vi "Find_All_References.vi"(6 "error in":errorcluster) -> (0 "error out":errorcluster, 1 "INI References":T1(array[cluster]), 2 "CTL References":T1(array[cluster]), 3 "VI References":T1(array[cluster]), 4 "Global References":T1(array[cluster]))   [LabVIEW 2021]
uses:
  Project_References_Global.vi
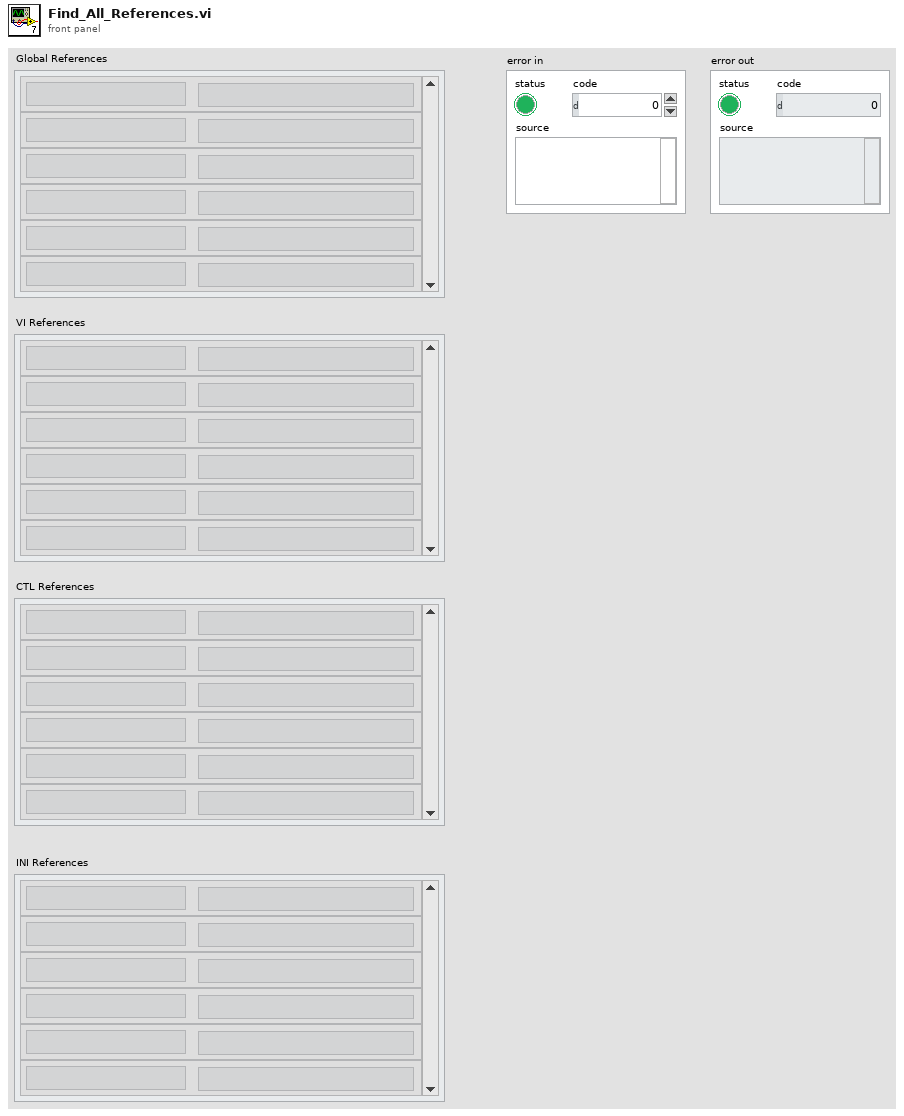
[diagram p1: front panel]
types:
  T1 = cluster{"VI Name":string, "String Path":string}[]
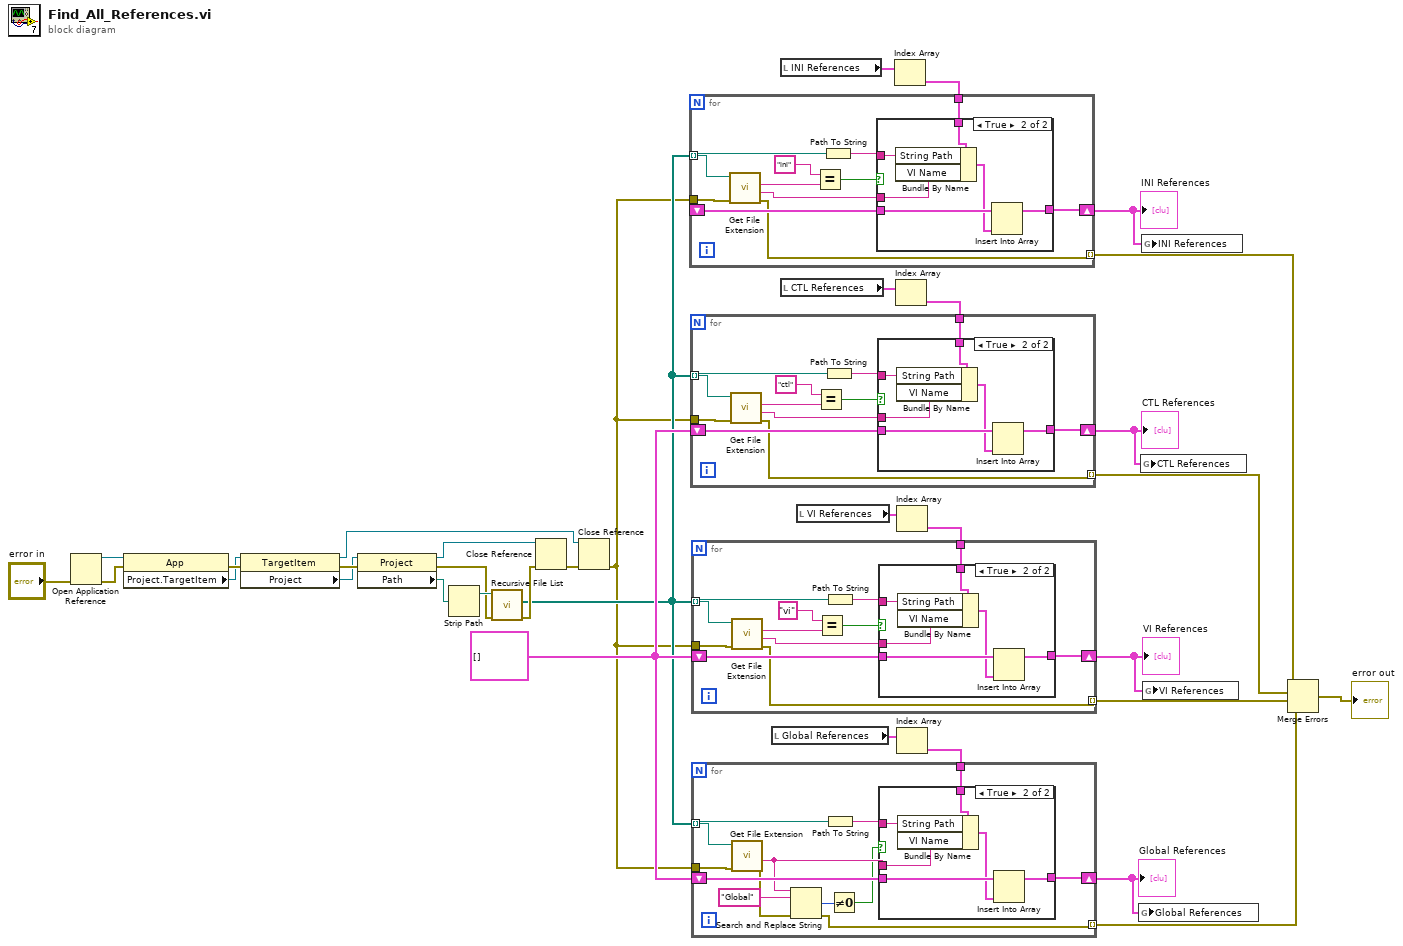
[diagram p0: block diagram]
diagram:
  w17 = T1 [] ("References")
  n1 = Open Application Reference(8:"error in") -> (0:w33:errorcluster, 3:w34:refnum<vi>)  [unwired: 3 in]
  n2 = property class="App"(reference=w34, error in=w33) -> (error out=w32:errorcluster, "Project.TargetItem"=w26:refnum<vi>)  [unwired: 1 out]
  n3 = property class="TargetItem"(reference=w26, error in=w32) -> (reference out=w27:refnum<vi>, error out=w31:errorcluster, "Project"=w30:refnum<vi>)
  n4 = property class="Project"(reference=w30, error in=w31) -> (reference out=w29:refnum<vi>, error out=w13:errorcluster, "Path"=w25:path)
  n5 = Strip Path(path=w25) -> (stripped path=w24:path)  [unwired: 1 out]
  n6 = call <vilib>:"Recursive File List.vi"("error in (no error)"=w13, "Folder Path"=w24) -> ("error out"=w12:errorcluster, "All Files in Dir"=w3:path[])  [unwired: 5 in, 3 out]
  n7 = Close Reference(reference=w29, error in (no error)=w12) -> (error out=w28:errorcluster)
  n8 = Close Reference(reference=w27, error in (no error)=w28) -> (error out=w2:errorcluster)
  n9 = local read "Global References"() -> (w20:T1)
  n10 = local read "INI References"() -> (w5:T1)
  n11 = local read "CTL References"() -> (w18:T1)
  n12 = local read "VI References"() -> (w23:T1)
  n13 = Index Array(array=w5) -> (element=w4:cluster{"VI Name":string, "String Path":string})  [unwired: 1 in]
  n14 = for {
    tunnel: w3 -> [w37] mode=indexing
    tunnel: w4 -> [w45]
    shift-right: [w39] -> w6
    shift-left: _ -> [w40]
    tunnel: w2 -> [w36]
    tunnel: [w35] -> w1 mode=indexing
    n15 = call <vilib>:"Get File Extension.vi"("error in (no error)"=w36, "file"=w37) -> ("error out"=w35:errorcluster, "filename without extension"=w41:string, "lowercase file extension"=w44:string)  [unwired: 5 in, 2 out]
    n16 = Equal?(x="ini", y=w44) -> (x = y?=w42:bool)
    n17 = Path To String(path=w37) -> (string=w38:string)
    n18 = case shown="True" w42 {
      tunnel: w45 -> [_ w52]
      tunnel: w41 -> [_ w51]
      tunnel: w38 -> [_ w50]
      tunnel: w40 -> [w46 w49]
      tunnel: [w46 w48] -> w39
      frame False {
      }
      frame True {
        n19 = Bundle By Name(cluster=w52, "String Path"=w50, "VI Name"=w51) -> (w47:cluster{"VI Name":string, "String Path":string})
        n20 = Insert Into Array(array=w49, new element=w47) -> (w48:T1)  [unwired: 1 in]
      }
    }
  }
  "INI References" <- w6
  n21 = Index Array(array=w18) -> (element=w19:cluster{"VI Name":string, "String Path":string})  [unwired: 1 in]
  n22 = for {
    tunnel: w3 -> [w55] mode=indexing
    tunnel: w19 -> [w63]
    shift-right: [w57] -> w16
    shift-left: w17 -> [w58]
    tunnel: w2 -> [w54]
    tunnel: [w53] -> w11 mode=indexing
    n23 = call <vilib>:"Get File Extension.vi"("error in (no error)"=w54, "file"=w55) -> ("error out"=w53:errorcluster, "filename without extension"=w59:string, "lowercase file extension"=w62:string)  [unwired: 5 in, 2 out]
    n24 = Equal?(x="ctl", y=w62) -> (x = y?=w60:bool)
    n25 = Path To String(path=w55) -> (string=w56:string)
    n26 = case shown="True" w60 {
      tunnel: w63 -> [_ w70]
      tunnel: w59 -> [_ w69]
      tunnel: w56 -> [_ w68]
      tunnel: w58 -> [w64 w67]
      tunnel: [w64 w66] -> w57
      frame False {
      }
      frame True {
        n27 = Bundle By Name(cluster=w70, "String Path"=w68, "VI Name"=w69) -> (w65:cluster{"VI Name":string, "String Path":string})
        n28 = Insert Into Array(array=w67, new element=w65) -> (w66:T1)  [unwired: 1 in]
      }
    }
  }
  "CTL References" <- w16
  n29 = Index Array(array=w23) -> (element=w22:cluster{"VI Name":string, "String Path":string})  [unwired: 1 in]
  n30 = for {
    tunnel: w3 -> [w73] mode=indexing
    tunnel: w22 -> [w81]
    shift-right: [w75] -> w15
    shift-left: w17 -> [w76]
    tunnel: w2 -> [w72]
    tunnel: [w71] -> w10 mode=indexing
    n31 = call <vilib>:"Get File Extension.vi"("error in (no error)"=w72, "file"=w73) -> ("error out"=w71:errorcluster, "filename without extension"=w77:string, "lowercase file extension"=w80:string)  [unwired: 5 in, 2 out]
    n32 = Equal?(x="vi", y=w80) -> (x = y?=w78:bool)
    n33 = Path To String(path=w73) -> (string=w74:string)
    n34 = case shown="True" w78 {
      tunnel: w81 -> [_ w88]
      tunnel: w77 -> [_ w87]
      tunnel: w74 -> [_ w86]
      tunnel: w76 -> [w82 w85]
      tunnel: [w82 w84] -> w75
      frame False {
      }
      frame True {
        n35 = Bundle By Name(cluster=w88, "String Path"=w86, "VI Name"=w87) -> (w83:cluster{"VI Name":string, "String Path":string})
        n36 = Insert Into Array(array=w85, new element=w83) -> (w84:T1)  [unwired: 1 in]
      }
    }
  }
  "VI References" <- w15
  n37 = Index Array(array=w20) -> (element=w21:cluster{"VI Name":string, "String Path":string})  [unwired: 1 in]
  n38 = for {
    tunnel: w3 -> [w96] mode=indexing
    tunnel: w21 -> [w100]
    shift-right: [w98] -> w14
    shift-left: w17 -> [w99]
    tunnel: w2 -> [w91]
    tunnel: [w89] -> w9 mode=indexing
    n39 = call <vilib>:"Get File Extension.vi"("error in (no error)"=w91, "file"=w96) -> ("error out"=w90:errorcluster, "filename without extension"=w95:string)  [unwired: 5 in, 3 out]
    n40 = Search and Replace String(input string=w95, search string="Global", error in=w90) -> (number of replacements=w93:i32, error out=w89:errorcluster)  [unwired: 5 in, 2 out]
    n41 = Path To String(path=w96) -> (string=w97:string)
    n42 = Not Equal To 0?(x=w93) -> (x != 0?=w92:bool)
    n43 = case shown="True" w92 {
      tunnel: w100 -> [_ w107]
      tunnel: w95 -> [_ w106]
      tunnel: w97 -> [_ w105]
      tunnel: w99 -> [w101 w104]
      tunnel: [w101 w103] -> w98
      frame False {
      }
      frame True {
        n44 = Bundle By Name(cluster=w107, "String Path"=w105, "VI Name"=w106) -> (w102:cluster{"VI Name":string, "String Path":string})
        n45 = Insert Into Array(array=w104, new element=w102) -> (w103:T1)  [unwired: 1 in]
      }
    }
  }
  "Global References" <- w14
  n46 = global write "Project_References_Global.vi" "Global References"(w14) -> ()
  n47 = global write "Project_References_Global.vi" "CTL References"(w16) -> ()
  n48 = global write "Project_References_Global.vi" "INI References"(w6) -> ()
  n49 = global write "Project_References_Global.vi" "VI References"(w15) -> ()
  n50 = Merge Errors(w1, w11, w10, w9) -> (→"error out":errorcluster)
